vi "GetPublicEvents.vi"(8 "error in (no error)":errorcluster, 11 "SMO":refnum<class "SMO.lvclass">) -> (0 "error out":errorcluster, 2 "Public Events":T1, 3 "SMO out":refnum<class "SMO.lvclass">)   [LabVIEW 2021, in "smo.lvlib" / "SMO.lvclass"]
uses:
  SMO.lvclass
  Typedefs/Public Events.ctl
  Typedefs/SMOState --Enum.ctl
  Typedefs/Reserve State--Enum.ctl
  SMO.lvclass/SMO.ctl
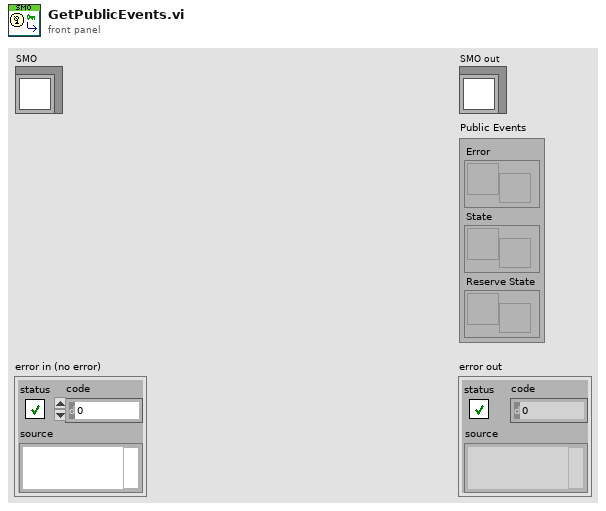
[diagram p1: front panel]
types:
  T1 = typedef "smo.lvlib/SMO.lvclass/Public Events.ctl" = cluster{"Error":refnum<user-event>, "State":refnum<user-event>, "Reserve State":refnum<user-event>}
  T2 = typedef "smo.lvlib/SMO.lvclass/PrivateData--Ref.ctl" = refnum<data-value>
  T3 = typedef "smo.lvlib/SMO.lvclass/PrivateData--Cluster.ctl" = cluster{"Parent Call":T4, "Registered Processes":T5[], "Sync Notifier":refnum<notifier>, "Process Error Notifier":refnum<notifier>, "Protected Events":T6, "Public Events":T1, "SMO State":T7, "[Attributes]":variant, "Launcher Close":refnum<notifier>, "Caller Watchdog":refnum<queue>, "Accessibility":T8, "NbStaticDependencies":u32}
  T4 = typedef "smo.lvlib/SMO.lvclass/Parent Call--Enum.ctl" = enum16{"Allows parent to run", "Does not request parent to run"}
  T5 = typedef "smo.lvlib/SMO.lvclass/RegisteredProcessData--Cluster.ctl" = cluster{"Name":string, "Static VI Ref":refnum<vi>, "Running":bool, "NotifierRef":u32}
  T6 = typedef "smo.lvlib/SMO.lvclass/Protected Events.ctl" = cluster{"StopProcesses":refnum<user-event>, "AbortProcesses":refnum<user-event>, "Config Changed":refnum<user-event>, "Dependency":refnum<user-event>}
  T7 = typedef "smo.lvlib/SMO.lvclass/SMOState --Enum.ctl" = enum16{"unknown", "Created", "Started", "Stopped"}
  T8 = typedef "smo.lvlib/SMO.lvclass/Accessibility--Cluster.ctl" = cluster{"Lock Key":string, "Reserve State":T9}
  T9 = typedef "smo.lvlib/SMO.lvclass/Reserve State--Enum.ctl" = enum16{"Unreserved", "Reserved", "Self-locked"}
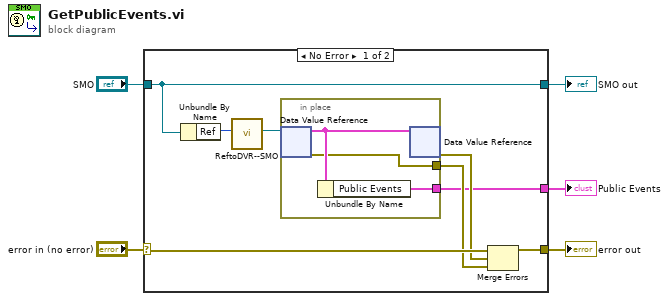
[diagram p0: block diagram]
diagram:
  n1 = case shown="No Error" "error in (no error)" {
    selector: "error in (no error)" -> [w13 w18]
    tunnel: [w12 w18] -> w4
    tunnel: [w6 w17] -> w2
    tunnel: "SMO" -> [w6 w17]
    tunnel: [w9 _] -> w1
    frame No Error {
      n2 = Unbundle By Name(w6) -> ("Ref"=w8:u32)
      n3 = call "ReftoDVR--SMO.vi"("Ref"=w8) -> ("Ref"=w7:T2)  [unwired: 10 in]
      n4 = in-place {
        in-place-border: [w16] -> w9
        in-place-border: [w14] -> w10
        n5 = in-place-dvr #1(w7) -> (w15:T3, w14:errorcluster)
        n6 = Unbundle By Name(w15) -> ("Public Events"=w16:T1)
        n7 = in-place-dvr #1(w15) -> (w11:errorcluster)  [unwired: 1 out]
      }
      n8 = Merge Errors(w13, w11, w10) -> (w12:errorcluster)
    }
    frame Error {
    }
  }
  "error out" <- w4
  "SMO out" <- w2
  "Public Events" <- w1
